vi "ZControlServo.vi"() -> ()   [LabVIEW 2014]
uses:
  <vilib>/Instr/_visa.llb/VISA Configure Serial Port (Instr).vi
panel:
  in  "position":u8(slide) scale=125.0..230.0
  in  "stop":bool
  in  "servo #":u8
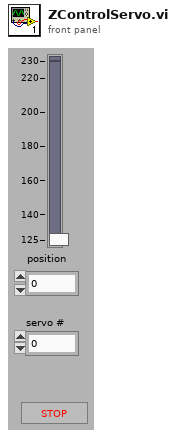
[diagram p1: front panel]
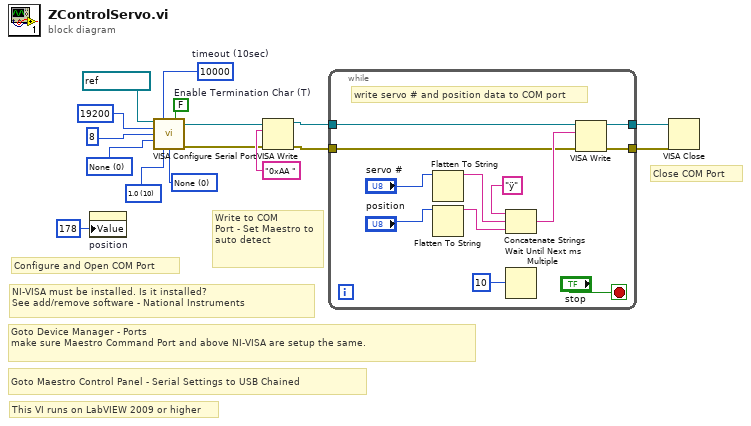
[diagram p0: block diagram]
diagram:
  w6 = u16 0 items=["None"=0, "XON/XOFF"=1, "RTS/CTS"=2, "DTR/DSR"=4] ("flow control")
  w7 = u16 10 items=["1.0"=10, "1.5"=15, "2.0"=20] ("stop bits")
  w8 = u16 0 items=["None", "Odd", "Even", "Mark", "Space"] ("parity")
  w12 = FALSE  # Enable Termination Char (T)
  w13 = u32 10000  # timeout (10sec)
  # "This VI runs on LabVIEW 2009 or higher"
  # "Goto Maestro Control Panel - Serial Settings to USB Chained"
  # "Close COM Port"
  # "Configure and Open COM Port"
  # "Goto Device Manager - Ports \nmake sure Maestro Command Port and above NI-VISA are setup the same."
  # "NI-VISA must be installed. Is it installed?\nSee add/remove software - National Instruments"
  # "Write to COM \nPort - Set Maestro to auto detect"
  n1 = property on="position" class="Slide (strict)"("Value"=u8 178 ("position")) -> ()  [unwired: 2 in, 2 out]
  n2 = call-poly "VISA Configure Serial Port"("VISA resource name"=refnum<visa-resource-name> "COM10", "timeout (10sec)"=w13, "Enable Termination\nChar (T)"=w12, "baud rate (9600)"=u32 19200 ("baud rate"), "data bits (8)"=u16 8 ("data bits"), "parity (0:none)"=w8, "stop bits (10: 1 bit)"=w7, "flow control (0:none)"=w6) -> ("VISA resource name out"=w4:refnum<visa-resource-name>, "error out"=w5:errorcluster)  [unwired: 1 in, 5 out]
  n3 = VISA Write(VISA resource name=w4, write buffer="0xAA ", error in (no error)=w5) -> (VISA resource name out=w15:refnum<visa-resource-name>, error out=w14:errorcluster)  [unwired: 1 out]
  n4 = while {
    tunnel: w15 -> [w23]
    tunnel: w14 -> [w22]
    tunnel: [w18] -> w3
    tunnel: [w17] -> w2
    stop <- "stop" stop-if-true
    # "write servo # and position data to COM port"
    n5 = Flatten To String(anything="servo #") -> (data string=w27:string)  [unwired: 1 in, 4 out]
    n6 = Flatten To String(anything="position") -> (data string=w26:string)  [unwired: 1 in, 4 out]
    n7 = Concatenate Strings("ÿ", w27, w26) -> (w25:string)
    n8 = Wait Until Next ms Multiple(millisecond multiple=10) -> ()  [unwired: 1 out]
    n9 = VISA Write(VISA resource name=w23, write buffer=w25, error in (no error)=w22) -> (VISA resource name out=w18:refnum<visa-resource-name>, error out=w17:errorcluster)  [unwired: 1 out]
  }
  n10 = VISA Close(VISA resource name=w3, error in (no error)=w2) -> ()  [unwired: 1 out]
